vi "Write.vi"(11 "MV":dbl(slide) scale=-100.0..100.0) -> ()   [LabVIEW 2018]
uses:
  <vilib>/DAQmx/write.llb/DAQmx Write (Digital 1D Bool NChan 1Samp 1Line).vi
  <vilib>/DAQmx/create/channels.llb/DAQmx Create Channel (DO-Digital Output).vi
  <vilib>/DAQmx/miscellaneous.llb/DAQmx Fill In Error Info.vi
panel:
  in  "stop":bool
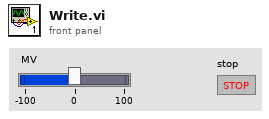
[diagram p1: front panel]
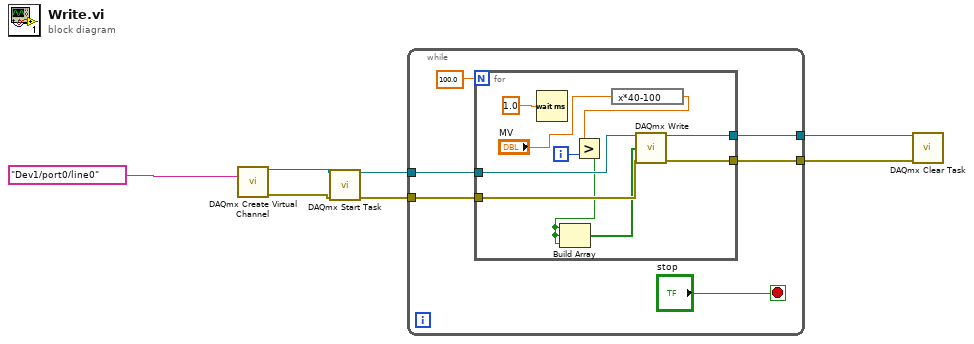
[diagram p0: block diagram]
diagram:
  n1 = call-poly <vilib>:"DAQmx Create Virtual Channel.vi"("lines"=tag "Dev1/port0/line0") -> ("task out"=w5:refnum<k21>, "error out"=w4:errorcluster)  [unwired: 13 in]
  n2 = call <vilib>:"DAQmx Start Task.vi"("task/channels in"=w5, "error in"=w4) -> ("task out"=w3:refnum<k21>, "error out"=w2:errorcluster)  [unwired: 12 in]
  n3 = while {
    tunnel: [w12] -> w7
    tunnel: [w11] -> w6
    tunnel: w3 -> [w10]
    tunnel: w2 -> [w9]
    stop <- "stop" stop-if-true
    n4 = for {
      N: 100.0 -> [_]
      tunnel: [w17] -> w12
      tunnel: [w21] -> w11
      tunnel: w10 -> [w20]
      tunnel: w9 -> [w19]
      i -> [w23]
      n5 = Wait (ms)(milliseconds to wait=1.0) -> ()  [unwired: 1 out]
      n6 = expression code="x*40-100"("MV") -> (w18:dbl)
      n7 = Greater?(x=w18, y=w23) -> (0:w15:bool)
      n8 = Build Array(w15, w15, w15) -> (w16:bool[])
      n9 = call-poly <vilib>:"DAQmx Write.vi"("task/channels in"=w20, "data"=w16, "error in"=w19) -> ("task out"=w17:refnum<k21>, "error out"=w21:errorcluster)  [unwired: 10 in, 1 out]
    }
  }
  n10 = call <vilib>:"DAQmx Clear Task.vi"("task in"=w7, "error in"=w6) -> ()  [unwired: 13 in, 1 out]
